vi "Set Limits on Configure Device.vi"(8 "error in (no error)":errorcluster, 9 "Max Beams":dbl, 10 "cluster":T1, 11 "Toggle 7.1 in":refnum<class "Toggle 7.1.lvclass">) -> (0 "error out":errorcluster, 3 "Toggle 7.1 out":refnum<class "Toggle 7.1.lvclass">)   [LabVIEW 2020, in "Toggle 7.1.lvclass"]
uses:
  Toggle 7.1.lvclass
  Controls/Configure decive refs cluster.ctl
  Controls/EFuse modes enum.ctl
  Controls/Set limit states.ctl
  <vilib>/Utility/miscctls.llb/LVMinMaxIncTypeDef.ctl
  <vilib>/Utility/miscctls.llb/LVOutOfRangeActionTypeDef.ctl
  Toggle 7.1.lvclass/Toggle 7.1.ctl
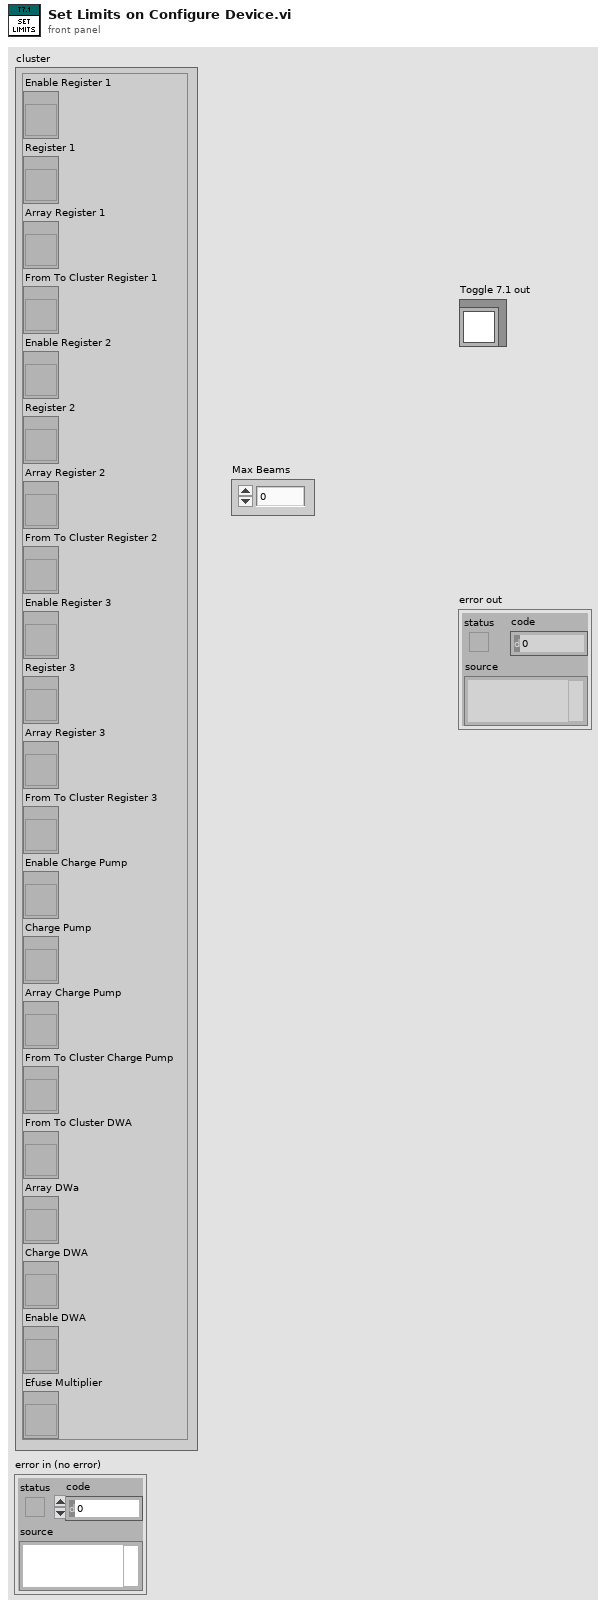
[diagram p1: front panel]
types:
  T1 = typedef "Toggle 7.1.lvclass/Configure decive refs cluster.ctl" = cluster{"Enable Register 1":refnum<vi>, "Register 1":refnum<vi>, "Array Register 1":refnum<vi>, "From To Cluster Register 1":refnum<vi>, "Enable Register 2":refnum<vi>, "Register 2":refnum<vi>, "Array Register 2":refnum<vi>, "From To Cluster Register 2":refnum<vi>, "Enable Register 3":refnum<vi>, "Register 3":refnum<vi>, "Array Register 3":refnum<vi>, "From To Cluster Register 3":refnum<vi>, "Enable Charge Pump":refnum<vi>, "Charge Pump":refnum<vi>, "Array Charge Pump":refnum<vi>, "From To Cluster Charge Pump":refnum<vi>, "From To Cluster DWA":refnum<vi>, "Array DWa":refnum<vi>, "Charge DWA":refnum<vi>, "Enable DWA":refnum<vi>, "Efuse Multiplier":refnum<vi>}
  T2 = typedef "Toggle 7.1.lvclass/Capacitor register.ctl" = cluster{"Register":u32, "Beam":dbl, "Trimmers":dbl[]}
  T3 = typedef "Toggle 7.1.lvclass/Set limit states.ctl" = enum16{"Reg 1", "Reg 2", "Reg 3", "DWA", "CP", "Efuse", "Info", "Done"}
  T4 = typedef "LVOutOfRangeActionTypeDef.ctl" = cluster{"Out of Range Action Minimum":u8, "Out of Range Action Maximum":u8, "Out of Range Action Increment":u8}
  T5 = typedef "LVMinMaxIncTypeDef.ctl" = cluster{"Minimum":dbl, "Maximum":dbl, "Increment":dbl}
  T6 = enum8{"Enabled", "Disabled", "Disabled and Grayed Out"}
  T7 = typedef "Toggle 7.1.lvclass/Parameter Cluster.ctl" = cluster{"Enable":bool, "Register Number":u32, "Use Array":bool, "Array":dbl[], "To From Cluster":cluster{"From":dbl, "To":dbl, "Step":dbl}}
  T8 = typedef "Toggle 7.1.lvclass/Charge Pump Information cluster.ctl" = cluster{"Min":dbl, "Max":dbl, "Step":dbl, "Default":dbl}
  T9 = typedef "Toggle 7.1.lvclass/EFuse modes enum.ctl" = enum16{"On", "Off", "Both On and Off"}
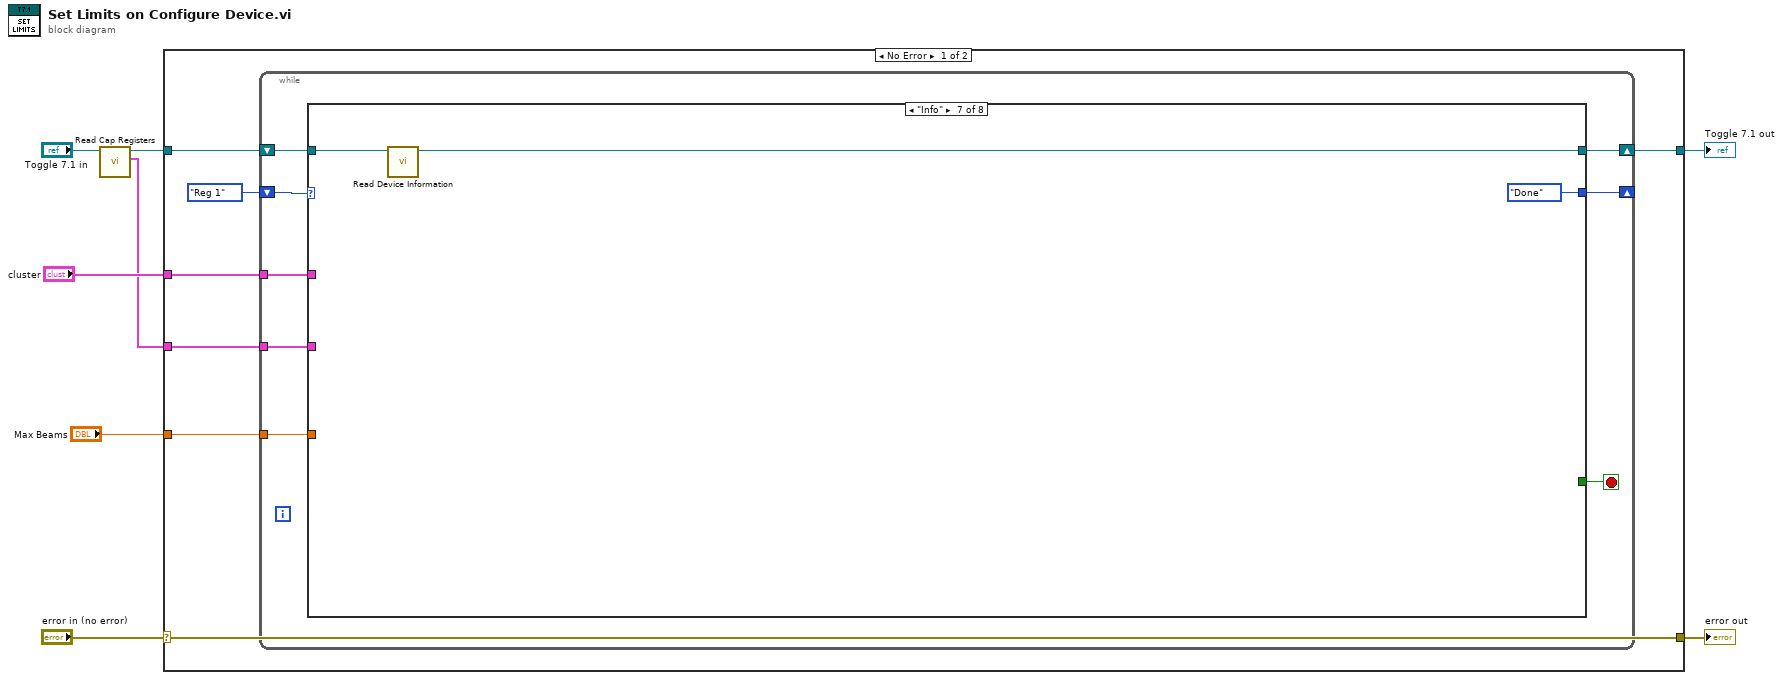
[diagram p0: block diagram]
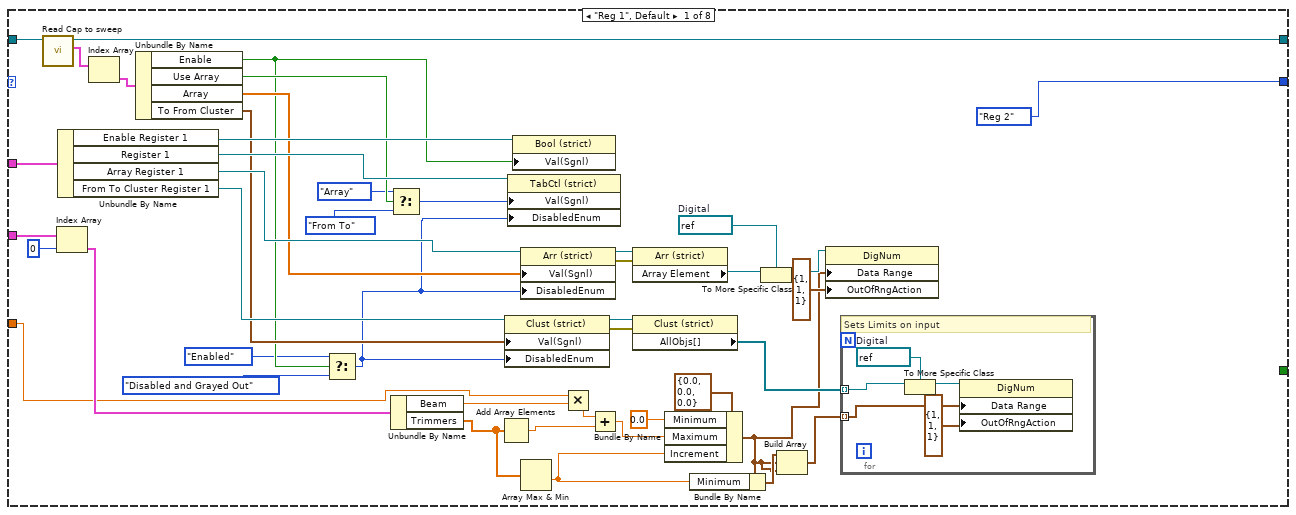
[diagram p2: hidden frame]
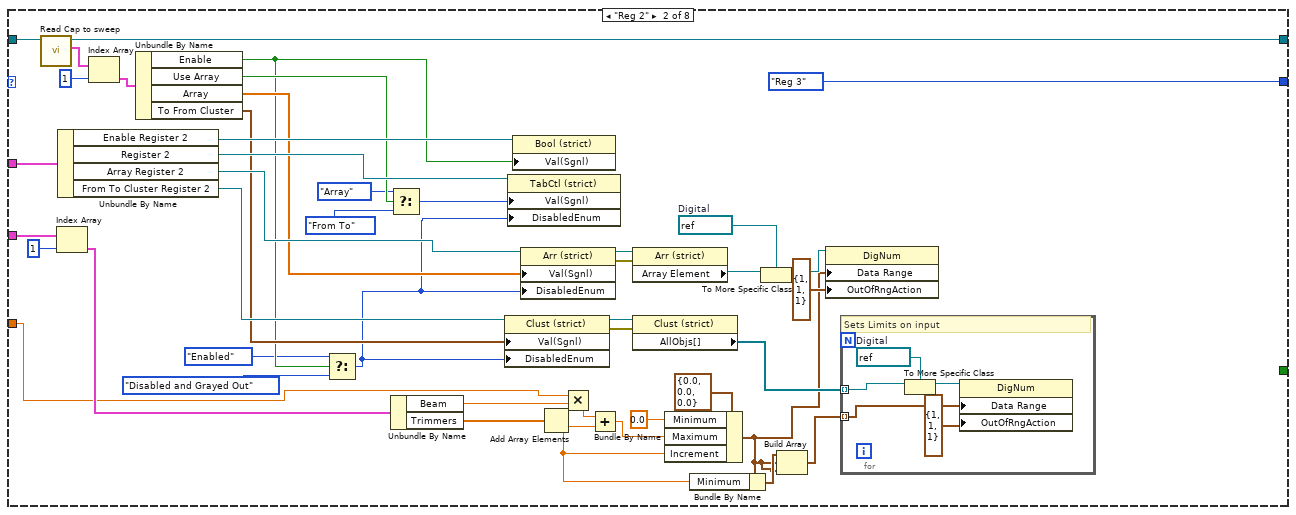
[diagram p3: hidden frame]
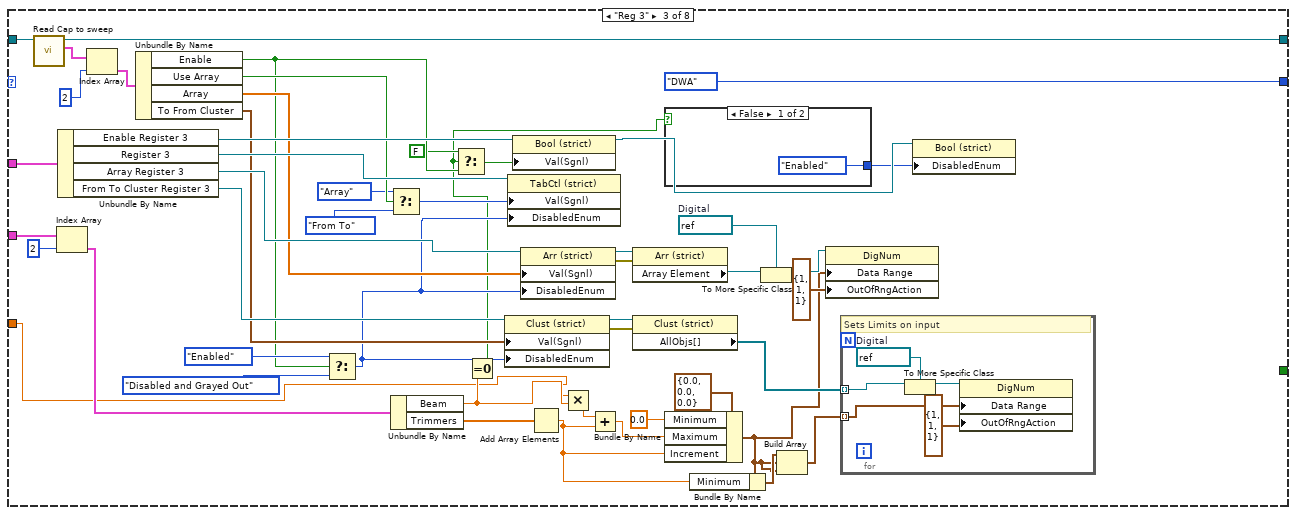
[diagram p4: hidden frame]
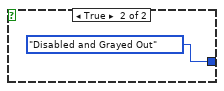
[diagram p5: hidden frame]
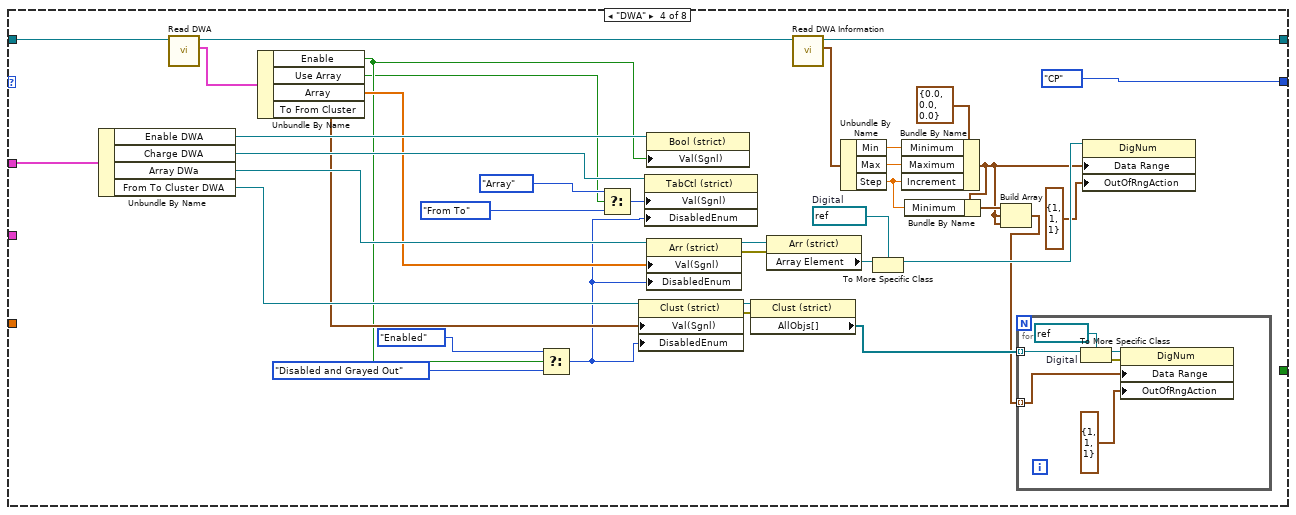
[diagram p6: hidden frame]
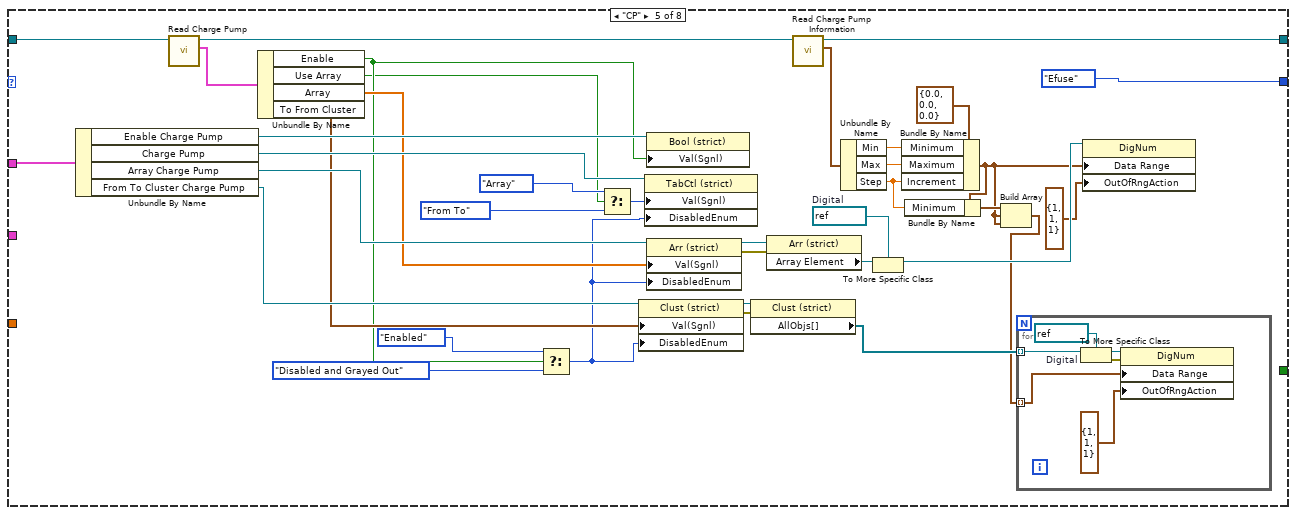
[diagram p7: hidden frame]
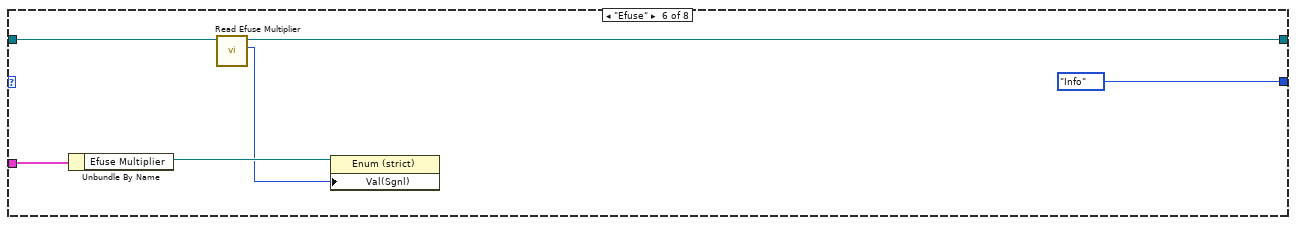
[diagram p8: hidden frame]
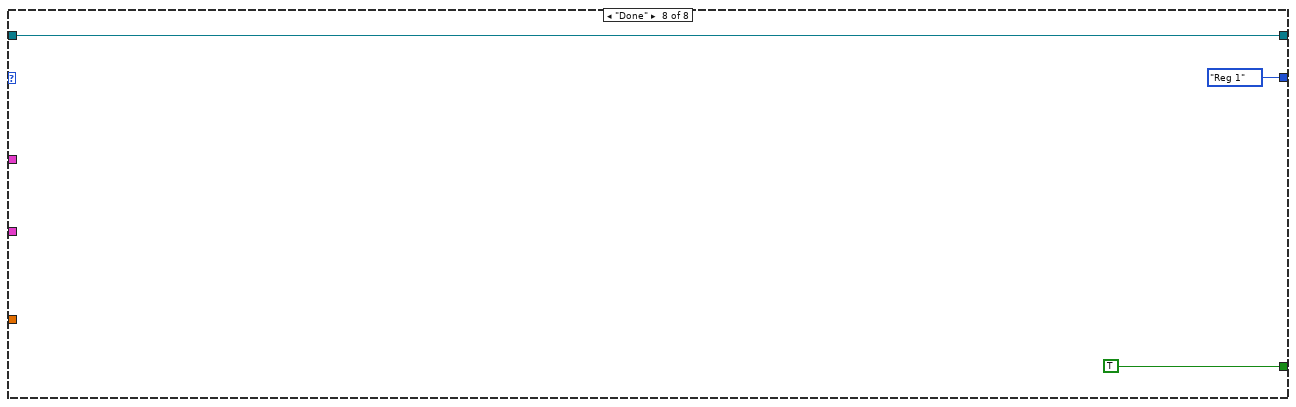
[diagram p9: hidden frame]
diagram:
  n1 = call-dynamic "Read Cap Registers.vi"("Toggle 6 in"="Toggle 7.1 in") -> ("Cap Registers"=w2:T2[], "Toggle 6 out"=w3:refnum<class "Toggle 7.1.lvclass">)  [unwired: 9 in]
  n2 = case shown="No Error" "error in (no error)" {
    selector: "error in (no error)" -> [w15 w277]
    tunnel: [w15 w277] -> w7
    tunnel: [w10 w276] -> w6
    tunnel: w3 -> [w14 w276]
    tunnel: "cluster" -> [w13 _]
    tunnel: w2 -> [w11 _]
    tunnel: "Max Beams" -> [w9 _]
    frame No Error {
      n3 = while {
        tunnel: w13 -> [w22]
        shift-right: [w20] -> w10
        shift-left: w14 -> [w23]
        shift-right: [w17] -> _
        shift-left: Set_limit_states."Reg 1" -> [w21]
        tunnel: w11 -> [w19]
        tunnel: w9 -> [w16]
        stop <- w18 stop-if-true
        n4 = case shown="\"Info\"" w21 {
          tunnel: w23 -> [w32 w80 w136 w214 w257 w268 w271 w274]
          tunnel: w22 -> [w67 w116 w170 w213 w256 w269 _ _]
          tunnel: [w31 w79 w135 w192 w235 w267 w270 w274] -> w20
          tunnel: [Set_limit_states."Reg 2" Set_limit_states."Reg 3" Set_limit_states."DWA" Set_limit_states."CP" Set_limit_states."Efuse" Set_limit_states."Info" Set_limit_states."Done" Set_limit_states."Reg 1"] -> w17
          tunnel: w19 -> [w52 w101 w156 _ _ _ _ _]
          tunnel: [_ _ _ _ _ _ _ TRUE] -> w18
          tunnel: w16 -> [w27 w73 w122 _ _ _ _ _]
          frame "Reg 1", Default {
            w37 = refnum<vi> refnum  # Digital
            n5 = call-dynamic "Read Cap to sweep.vi"("Toggle 6 in"=w32) -> ("Cap to sweep"=w30:T7[], "Toggle 6 out"=w31:refnum<class "Toggle 7.1.lvclass">)  [unwired: 9 in]
            n6 = Index Array(array=w52, index=0) -> (element=w50:T2)
            n7 = Unbundle By Name(w67) -> ("Enable Register 1"=w66:refnum<vi>, "Register 1"=w65:refnum<vi>, "Array Register 1"=w60:refnum<vi>, "From To Cluster Register 1"=w58:refnum<vi>)
            n8 = Index Array(array=w30) -> (element=w29:T7)  [unwired: 1 in]
            n9 = Unbundle By Name(w29) -> ("Enable"=w56:bool, "Use Array"=w63:bool, "Array"=w59:dbl[], "To From Cluster"=w57:cluster{"From":dbl, "To":dbl, "Step":dbl})
            n10 = Select(t=T6."Enabled" ("Disabled"), s=w56, f=T6."Disabled and Grayed Out" ("Disabled")) -> (s? t:f=w53:T6)
            n11 = Select(t=enum32{"From To", "Array"}."Array", s=w63, f=enum32{"From To", "Array"}."From To" ("Value (Signaling)")) -> (s? t:f=w64:enum32{"From To", "Array"})
            n12 = Unbundle By Name(w50) -> ("Beam"=w46:dbl, "Trimmers"=w25:dbl[])
            n13 = Add Array Elements(numeric array=w25) -> (sum=w26:dbl)
            n14 = property class="Clust (strict)"(reference=w58, "Val(Sgnl)"=w57, "DisabledEnum"=w53) -> (reference out=w49:refnum<vi>, error out=w48:errorcluster)  [unwired: 1 in]
            n15 = property class="TabCtl (strict)"(reference=w65, "Val(Sgnl)"=w64, "DisabledEnum"=w53) -> ()  [unwired: 1 in, 2 out]
            n16 = property class="Bool (strict)"(reference=w66, "Val(Sgnl)"=w56) -> ()  [unwired: 1 in, 2 out]
            n17 = property class="Arr (strict)"(reference=w60, "Val(Sgnl)"=w59, "DisabledEnum"=w53) -> (reference out=w40:refnum<vi>, error out=w39:errorcluster)  [unwired: 1 in]
            n18 = Array Max & Min(array=w25) -> (min value=w24:dbl)  [unwired: 3 out]
            n19 = Multiply(x=w27, y=w46) -> (x*y=w43:dbl)
            n20 = Add(x=w43, y=w26) -> (x+y=w42:dbl)
            n21 = property class="Arr (strict)"(reference=w40, error in=w39) -> ("Array Element"=w38:refnum<vi>)  [unwired: 2 out]
            n22 = property class="Clust (strict)"(reference=w49, error in=w48) -> ("AllObjs[]"=w47:refnum<vi>[])  [unwired: 2 out]
            n23 = Bundle By Name(cluster=T5 {"Minimum"=0.0, "Maximum"=0.0, "Increment"=0.0} ("Data Entry Limits"), "Minimum"=0.0, "Maximum"=w42, "Increment"=w24) -> (w33:T5)
            n24 = Bundle By Name(cluster=w33, "Minimum"=w24) -> (w34:T5)
            n25 = To More Specific Class(target class=w37, reference=w38) -> (specific class reference=w36:refnum<vi>)  [unwired: 1 in, 1 out]
            n26 = Build Array(w34, w33, w33) -> (w41:T5[])
            n27 = property class="DigNum"(reference=w36, "Data Range"=w33, "OutOfRngAction"=T4 {"Out of Range Action Minimum"=1, "Out of Range Action Maximum"=1, "Out of Range Action Increment"=1} ("Response to Value Outside Limits")) -> ()  [unwired: 1 in, 2 out]
            n28 = for {
              tunnel: w47 -> [w71] mode=indexing
              tunnel: w41 -> [w69] mode=indexing
              w72 = refnum<vi> refnum  # Digital
              # "Sets Limits on input"
              n29 = To More Specific Class(target class=w72, reference=w71) -> (specific class reference=w70:refnum<vi>)  [unwired: 1 in, 1 out]
              n30 = property class="DigNum"(reference=w70, "Data Range"=w69, "OutOfRngAction"=T4 {"Out of Range Action Minimum"=1, "Out of Range Action Maximum"=1, "Out of Range Action Increment"=1} ("Response to Value Outside Limits")) -> ()  [unwired: 1 in, 2 out]
            }
          }
          frame "Reg 2" {
            w85 = refnum<vi> refnum  # Digital
            n31 = call-dynamic "Read Cap to sweep.vi"("Toggle 6 in"=w80) -> ("Cap to sweep"=w78:T7[], "Toggle 6 out"=w79:refnum<class "Toggle 7.1.lvclass">)  [unwired: 9 in]
            n32 = Index Array(array=w101, index=1) -> (element=w99:T2)
            n33 = Unbundle By Name(w116) -> ("Enable Register 2"=w115:refnum<vi>, "Register 2"=w114:refnum<vi>, "Array Register 2"=w109:refnum<vi>, "From To Cluster Register 2"=w107:refnum<vi>)
            n34 = Index Array(array=w78, index=1) -> (element=w76:T7)
            n35 = Unbundle By Name(w76) -> ("Enable"=w105:bool, "Use Array"=w112:bool, "Array"=w108:dbl[], "To From Cluster"=w106:cluster{"From":dbl, "To":dbl, "Step":dbl})
            n36 = Select(t=T6."Enabled" ("Disabled"), s=w105, f=T6."Disabled and Grayed Out" ("Disabled")) -> (s? t:f=w102:T6)
            n37 = Select(t=enum32{"From To", "Array"}."Array", s=w112, f=enum32{"From To", "Array"}."From To" ("Value (Signaling)")) -> (s? t:f=w113:enum32{"From To", "Array"})
            n38 = Unbundle By Name(w99) -> ("Beam"=w95:dbl, "Trimmers"=w90:dbl[])
            n39 = property class="Clust (strict)"(reference=w107, "Val(Sgnl)"=w106, "DisabledEnum"=w102) -> (reference out=w98:refnum<vi>, error out=w97:errorcluster)  [unwired: 1 in]
            n40 = property class="TabCtl (strict)"(reference=w114, "Val(Sgnl)"=w113, "DisabledEnum"=w102) -> ()  [unwired: 1 in, 2 out]
            n41 = property class="Bool (strict)"(reference=w115, "Val(Sgnl)"=w105) -> ()  [unwired: 1 in, 2 out]
            n42 = property class="Arr (strict)"(reference=w109, "Val(Sgnl)"=w108, "DisabledEnum"=w102) -> (reference out=w88:refnum<vi>, error out=w87:errorcluster)  [unwired: 1 in]
            n43 = Add Array Elements(numeric array=w90) -> (sum=w74:dbl)
            n44 = Multiply(x=w73, y=w95) -> (x*y=w92:dbl)
            n45 = Add(x=w92, y=w74) -> (x+y=w91:dbl)
            n46 = property class="Arr (strict)"(reference=w88, error in=w87) -> ("Array Element"=w86:refnum<vi>)  [unwired: 2 out]
            n47 = property class="Clust (strict)"(reference=w98, error in=w97) -> ("AllObjs[]"=w96:refnum<vi>[])  [unwired: 2 out]
            n48 = Bundle By Name(cluster=T5 {"Minimum"=0.0, "Maximum"=0.0, "Increment"=0.0} ("Data Entry Limits"), "Minimum"=0.0, "Maximum"=w91, "Increment"=w74) -> (w81:T5)
            n49 = Bundle By Name(cluster=w81, "Minimum"=w74) -> (w82:T5)
            n50 = To More Specific Class(target class=w85, reference=w86) -> (specific class reference=w84:refnum<vi>)  [unwired: 1 in, 1 out]
            n51 = Build Array(w82, w81, w81) -> (w89:T5[])
            n52 = property class="DigNum"(reference=w84, "Data Range"=w81, "OutOfRngAction"=T4 {"Out of Range Action Minimum"=1, "Out of Range Action Maximum"=1, "Out of Range Action Increment"=1} ("Response to Value Outside Limits")) -> ()  [unwired: 1 in, 2 out]
            n53 = for {
              tunnel: w96 -> [w120] mode=indexing
              tunnel: w89 -> [w118] mode=indexing
              w121 = refnum<vi> refnum  # Digital
              # "Sets Limits on input"
              n54 = To More Specific Class(target class=w121, reference=w120) -> (specific class reference=w119:refnum<vi>)  [unwired: 1 in, 1 out]
              n55 = property class="DigNum"(reference=w119, "Data Range"=w118, "OutOfRngAction"=T4 {"Out of Range Action Minimum"=1, "Out of Range Action Maximum"=1, "Out of Range Action Increment"=1} ("Response to Value Outside Limits")) -> ()  [unwired: 1 in, 2 out]
            }
          }
          frame "Reg 3" {
            w141 = refnum<vi> refnum  # Digital
            n56 = call-dynamic "Read Cap to sweep.vi"("Toggle 6 in"=w136) -> ("Cap to sweep"=w134:T7[], "Toggle 6 out"=w135:refnum<class "Toggle 7.1.lvclass">)  [unwired: 9 in]
            n57 = Index Array(array=w156, index=2) -> (element=w154:T2)
            n58 = Unbundle By Name(w170) -> ("Enable Register 3"=w169:refnum<vi>, "Register 3"=w168:refnum<vi>, "Array Register 3"=w163:refnum<vi>, "From To Cluster Register 3"=w161:refnum<vi>)
            n59 = Index Array(array=w134, index=2) -> (element=w133:T7)
            n60 = Unbundle By Name(w133) -> ("Enable"=w127:bool, "Use Array"=w166:bool, "Array"=w162:dbl[], "To From Cluster"=w160:cluster{"From":dbl, "To":dbl, "Step":dbl})
            n61 = Select(t=T6."Enabled" ("Disabled"), s=w127, f=T6."Disabled and Grayed Out" ("Disabled")) -> (s? t:f=w157:T6)
            n62 = Select(t=enum32{"From To", "Array"}."Array", s=w166, f=enum32{"From To", "Array"}."From To" ("Value (Signaling)")) -> (s? t:f=w167:enum32{"From To", "Array"})
            n63 = Unbundle By Name(w154) -> ("Beam"=w129:dbl, "Trimmers"=w146:dbl[])
            n64 = Equal To 0?(x=w129) -> (x = 0?=w125:bool)
            n65 = Select(t=FALSE, s=w125, f=w127) -> (s? t:f=w128:bool)
            n66 = property class="Clust (strict)"(reference=w161, "Val(Sgnl)"=w160, "DisabledEnum"=w157) -> (reference out=w153:refnum<vi>, error out=w152:errorcluster)  [unwired: 1 in]
            n67 = property class="TabCtl (strict)"(reference=w168, "Val(Sgnl)"=w167, "DisabledEnum"=w157) -> ()  [unwired: 1 in, 2 out]
            n68 = property class="Bool (strict)"(reference=w169, "Val(Sgnl)"=w128) -> (reference out=w124:refnum<vi>)  [unwired: 1 in, 1 out]
            n69 = property class="Arr (strict)"(reference=w163, "Val(Sgnl)"=w162, "DisabledEnum"=w157) -> (reference out=w144:refnum<vi>, error out=w143:errorcluster)  [unwired: 1 in]
            n70 = Add Array Elements(numeric array=w146) -> (sum=w130:dbl)
            n71 = Multiply(x=w122, y=w129) -> (x*y=w148:dbl)
            n72 = Add(x=w148, y=w130) -> (x+y=w147:dbl)
            n73 = property class="Arr (strict)"(reference=w144, error in=w143) -> ("Array Element"=w142:refnum<vi>)  [unwired: 2 out]
            n74 = property class="Clust (strict)"(reference=w153, error in=w152) -> ("AllObjs[]"=w151:refnum<vi>[])  [unwired: 2 out]
            n75 = case shown="False" w125 {
              tunnel: [T6."Enabled" ("Disabled") T6."Disabled and Grayed Out" ("Disabled")] -> w123
              frame False {
              }
              frame True {
              }
            }
            n76 = Bundle By Name(cluster=T5 {"Minimum"=0.0, "Maximum"=0.0, "Increment"=0.0} ("Data Entry Limits"), "Minimum"=0.0, "Maximum"=w147, "Increment"=w130) -> (w137:T5)
            n77 = Bundle By Name(cluster=w137, "Minimum"=w130) -> (w138:T5)
            n78 = To More Specific Class(target class=w141, reference=w142) -> (specific class reference=w140:refnum<vi>)  [unwired: 1 in, 1 out]
            n79 = Build Array(w138, w137, w137) -> (w145:T5[])
            n80 = property class="DigNum"(reference=w140, "Data Range"=w137, "OutOfRngAction"=T4 {"Out of Range Action Minimum"=1, "Out of Range Action Maximum"=1, "Out of Range Action Increment"=1} ("Response to Value Outside Limits")) -> ()  [unwired: 1 in, 2 out]
            n81 = for {
              tunnel: w151 -> [w176] mode=indexing
              tunnel: w145 -> [w174] mode=indexing
              w177 = refnum<vi> refnum  # Digital
              # "Sets Limits on input"
              n82 = To More Specific Class(target class=w177, reference=w176) -> (specific class reference=w175:refnum<vi>)  [unwired: 1 in, 1 out]
              n83 = property class="DigNum"(reference=w175, "Data Range"=w174, "OutOfRngAction"=T4 {"Out of Range Action Minimum"=1, "Out of Range Action Maximum"=1, "Out of Range Action Increment"=1} ("Response to Value Outside Limits")) -> ()  [unwired: 1 in, 2 out]
            }
            n84 = property class="Bool (strict)"(reference=w124, "DisabledEnum"=w123) -> ()  [unwired: 1 in, 2 out]
          }
          frame "DWA" {
            w195 = refnum<vi> refnum  # Digital
            n85 = Unbundle By Name(w213) -> ("Enable DWA"=w211:refnum<vi>, "Charge DWA"=w210:refnum<vi>, "Array DWa"=w206:refnum<vi>, "From To Cluster DWA"=w204:refnum<vi>)
            n86 = call "Read DWA.vi"("Toggle 7.1 in"=w214) -> ("Parameter Cluster"=w212:T7, "Toggle 7.1 out"=w193:refnum<class "Toggle 7.1.lvclass">)  [unwired: 9 in]
            n87 = Unbundle By Name(w212) -> ("Enable"=w202:bool, "Use Array"=w178:bool, "Array"=w205:dbl[], "To From Cluster"=w203:cluster{"From":dbl, "To":dbl, "Step":dbl})
            n88 = Select(t=T6."Enabled" ("Disabled"), s=w202, f=T6."Disabled and Grayed Out") -> (s? t:f=w199:T6)
            n89 = Select(t=enum32{"From To", "Array"}."Array" ("Value (Signaling)"), s=w178, f=enum32{"From To", "Array"}."From To") -> (s? t:f=w208:enum32{"From To", "Array"})
            n90 = property class="Clust (strict)"(reference=w204, "Val(Sgnl)"=w203, "DisabledEnum"=w199) -> (reference out=w187:refnum<vi>, error out=w186:errorcluster)  [unwired: 1 in]
            n91 = property class="TabCtl (strict)"(reference=w210, "Val(Sgnl)"=w208, "DisabledEnum"=w199) -> ()  [unwired: 1 in, 2 out]
            n92 = property class="Bool (strict)"(reference=w211, "Val(Sgnl)"=w202) -> ()  [unwired: 1 in, 2 out]
            n93 = property class="Arr (strict)"(reference=w206, "Val(Sgnl)"=w205, "DisabledEnum"=w199) -> (reference out=w198:refnum<vi>, error out=w197:errorcluster)  [unwired: 1 in]
            n94 = property class="Clust (strict)"(reference=w187, error in=w186) -> ("AllObjs[]"=w185:refnum<vi>[])  [unwired: 2 out]
            n95 = property class="Arr (strict)"(reference=w198, error in=w197) -> ("Array Element"=w196:refnum<vi>)  [unwired: 2 out]
            n96 = call "Read DWA Information.vi"("Toggle 7.1 in"=w193) -> ("DWA Information"=w190:T8, "Toggle 7.1 out"=w192:refnum<class "Toggle 7.1.lvclass">)  [unwired: 9 in]
            n97 = Unbundle By Name(w190) -> ("Min"=w189:dbl, "Max"=w188:dbl, "Step"=w184:dbl)
            n98 = To More Specific Class(target class=w195, reference=w196) -> (specific class reference=w194:refnum<vi>)  [unwired: 1 in, 1 out]
            n99 = Bundle By Name(cluster=T5 {"Minimum"=0.0, "Maximum"=0.0, "Increment"=0.0} ("Data Entry Limits"), "Minimum"=w189, "Maximum"=w188, "Increment"=w184) -> (w182:T5)
            n100 = Bundle By Name(cluster=w182, "Minimum"=w184) -> (w183:T5)
            n101 = Build Array(w183, w182, w182) -> (w181:T5[])
            n102 = for {
              tunnel: w185 -> [w220] mode=indexing
              tunnel: w181 -> [w216] mode=indexing
              w219 = refnum<vi> refnum  # Digital
              n103 = To More Specific Class(target class=w219, reference=w220) -> (specific class reference=w218:refnum<vi>, error out=w217:errorcluster)  [unwired: 1 in]
              n104 = property class="DigNum"(reference=w218, error in=w217, "Data Range"=w216, "OutOfRngAction"=T4 {"Out of Range Action Minimum"=1, "Out of Range Action Maximum"=1, "Out of Range Action Increment"=1} ("Response to Value Outside Limits")) -> ()  [unwired: 2 out]
            }
            n105 = property class="DigNum"(reference=w194, "Data Range"=w182, "OutOfRngAction"=T4 {"Out of Range Action Minimum"=1, "Out of Range Action Maximum"=1, "Out of Range Action Increment"=1} ("Response to Value Outside Limits")) -> ()  [unwired: 1 in, 2 out]
          }
          frame "CP" {
            w238 = refnum<vi> refnum  # Digital
            n106 = Unbundle By Name(w256) -> ("Enable Charge Pump"=w254:refnum<vi>, "Charge Pump"=w253:refnum<vi>, "Array Charge Pump"=w249:refnum<vi>, "From To Cluster Charge Pump"=w247:refnum<vi>)
            n107 = call-dynamic "Read Charge Pump.vi"("Toggle 7.1 in"=w257) -> ("Parameter Cluster"=w255:T7, "Toggle 7.1 out"=w236:refnum<class "Toggle 7.1.lvclass">)  [unwired: 8 in, 1 out]
            n108 = Unbundle By Name(w255) -> ("Enable"=w245:bool, "Use Array"=w221:bool, "Array"=w248:dbl[], "To From Cluster"=w246:cluster{"From":dbl, "To":dbl, "Step":dbl})
            n109 = Select(t=T6."Enabled" ("Disabled"), s=w245, f=T6."Disabled and Grayed Out") -> (s? t:f=w242:T6)
            n110 = Select(t=enum32{"From To", "Array"}."Array" ("Value (Signaling)"), s=w221, f=enum32{"From To", "Array"}."From To") -> (s? t:f=w251:enum32{"From To", "Array"})
            n111 = property class="Clust (strict)"(reference=w247, "Val(Sgnl)"=w246, "DisabledEnum"=w242) -> (reference out=w230:refnum<vi>, error out=w229:errorcluster)  [unwired: 1 in]
            n112 = property class="TabCtl (strict)"(reference=w253, "Val(Sgnl)"=w251, "DisabledEnum"=w242) -> ()  [unwired: 1 in, 2 out]
            n113 = property class="Bool (strict)"(reference=w254, "Val(Sgnl)"=w245) -> ()  [unwired: 1 in, 2 out]
            n114 = property class="Arr (strict)"(reference=w249, "Val(Sgnl)"=w248, "DisabledEnum"=w242) -> (reference out=w241:refnum<vi>, error out=w240:errorcluster)  [unwired: 1 in]
            n115 = property class="Clust (strict)"(reference=w230, error in=w229) -> ("AllObjs[]"=w228:refnum<vi>[])  [unwired: 2 out]
            n116 = property class="Arr (strict)"(reference=w241, error in=w240) -> ("Array Element"=w239:refnum<vi>)  [unwired: 2 out]
            n117 = call-dynamic "Read Charge Pump Information.vi"("Toggle 6 in"=w236) -> ("Charge Pump Information"=w233:T8, "Toggle 6 out"=w235:refnum<class "Toggle 7.1.lvclass">)  [unwired: 9 in]
            n118 = Unbundle By Name(w233) -> ("Min"=w232:dbl, "Max"=w231:dbl, "Step"=w227:dbl)
            n119 = To More Specific Class(target class=w238, reference=w239) -> (specific class reference=w237:refnum<vi>)  [unwired: 1 in, 1 out]
            n120 = Bundle By Name(cluster=T5 {"Minimum"=0.0, "Maximum"=0.0, "Increment"=0.0} ("Data Entry Limits"), "Minimum"=w232, "Maximum"=w231, "Increment"=w227) -> (w225:T5)
            n121 = Bundle By Name(cluster=w225, "Minimum"=w227) -> (w226:T5)
            n122 = Build Array(w226, w225, w225) -> (w224:T5[])
            n123 = for {
              tunnel: w228 -> [w263] mode=indexing
              tunnel: w224 -> [w259] mode=indexing
              w262 = refnum<vi> refnum  # Digital
              n124 = To More Specific Class(target class=w262, reference=w263) -> (specific class reference=w261:refnum<vi>, error out=w260:errorcluster)  [unwired: 1 in]
              n125 = property class="DigNum"(reference=w261, error in=w260, "Data Range"=w259, "OutOfRngAction"=T4 {"Out of Range Action Minimum"=1, "Out of Range Action Maximum"=1, "Out of Range Action Increment"=1} ("Response to Value Outside Limits")) -> ()  [unwired: 2 out]
            }
            n126 = property class="DigNum"(reference=w237, "Data Range"=w225, "OutOfRngAction"=T4 {"Out of Range Action Minimum"=1, "Out of Range Action Maximum"=1, "Out of Range Action Increment"=1} ("Response to Value Outside Limits")) -> ()  [unwired: 1 in, 2 out]
          }
          frame "Efuse" {
            n127 = Unbundle By Name(w269) -> ("Efuse Multiplier"=w266:refnum<vi>)
            n128 = call-dynamic "Read Efuse Multiplier.vi"("Toggle 6 in"=w268) -> ("Efuse Multiplier"=w265:T9, "Toggle 6 out"=w267:refnum<class "Toggle 7.1.lvclass">)  [unwired: 9 in]
            n129 = property class="Enum (strict)"(reference=w266, "Val(Sgnl)"=w265) -> ()  [unwired: 1 in, 2 out]
          }
          frame "Info" {
            n130 = call-dynamic "Read Device Information.vi"("Device in"=w271) -> ("Device out"=w270:refnum<class "Toggle 7.1.lvclass">)  [unwired: 8 in, 2 out]
          }
          frame "Done" {
          }
        }
      }
    }
    frame Error {
    }
  }
  "error out" <- w7
  "Toggle 7.1 out" <- w6
